vi "Chain2_bak.vi"(7 "Name (\"\" to Use UUID)":string="CSM-Module") -> ()   [LabVIEW 2017, in "CSM-Testcase.lvlib"]
doc: "Creates a template for a CSM module without a user interface.\n\n> [!NOTE] CSM Name Rules\n> - The CSM module name must be unique to avoid entering the \"Critical Error\" state.\n> - If the input is \"\", a UUID will be used as the module name. This module will operate in independent mode and will not be listed in the module list.\n> - If the input ends with '#', the module will run in work mode. Modules with the same name will share the same message queue. External messages will be handled by the idle module.\n\n> [!NOTE] CSM Initialization State\n> - The default value is \"Macro: Initialize\", consistent with the JKISM state machine.\n> - This state is typically not modified and is provided to facilitate external programmatic changes to the initialization state.\n\n\n-- <b>Controls</b> --\n- <b>Name (\"\" to Use UUID)</b>: CSM Module Name\n- <b>Init State(\"Macro: Initialize\")</b>: Initialization State, default is \"Macro: Initialize\""
uses:
  CSM-Testcase.lvlib
  250f9197-eaab-42aa-85f4-d19595f3ef40.vi
  b1f9a1d7-2f6f-40c5-bed8-42b286b8eb3f.vi
  e695532a-dccc-48b0-b567-f6fcd461bdfb.vi
  src/user.lib/_NEVSTOP/Communicable State Machine(CSM)/AdvanceAPI/CSM - Revert Arguments-Safe String.vi
  src/user.lib/_NEVSTOP/Communicable State Machine(CSM)/AdvanceAPI/CSM - Make String Arguments Safe.vi
  src/user.lib/_NEVSTOP/Communicable State Machine(CSM)/AdvanceAPI/CSM - Break Down Multiple States String.vi
  src/user.lib/_NEVSTOP/Communicable State Machine(CSM)/AdvanceAPI/CSM - Keywords.vi
  src/user.lib/_NEVSTOP/Communicable State Machine(CSM)/_Shared/Trim Single-line Text.vi
  Global-TestcaseCSM.vi
  src/user.lib/_NEVSTOP/Communicable State Machine(CSM)/_Polymophic/Build No-Reply Asynchronous Message with Arguments.vi
  src/user.lib/_NEVSTOP/Communicable State Machine(CSM)/_Polymophic/Build Asynchronous Message with Arguments.vi
  src/user.lib/_NEVSTOP/Communicable State Machine(CSM)/_Polymophic/Build Register Status Message.vi
  src/user.lib/_NEVSTOP/Communicable State Machine(CSM)/_Polymophic/Build Unregister Status Message.vi
  src/user.lib/_NEVSTOP/Communicable State Machine(CSM)/Communicable State Machine.lvlib
panel:
  out "Error Occurred":errorcluster
  out "State History":string
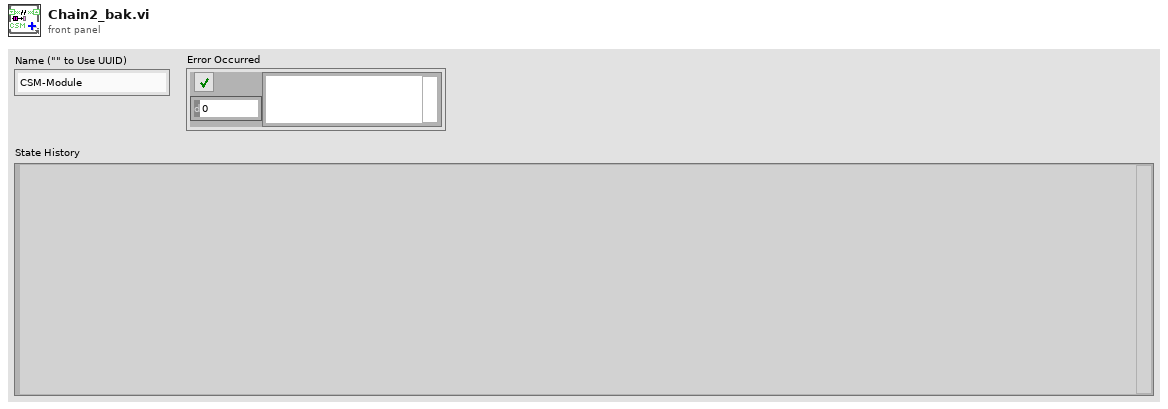
[diagram p1: front panel]
types:
  T1 = cluster{"Arguments":string, "Response":string, "error":errorcluster}
  T2 = enum32{"Invalid", "Standard", "Closed", "Hidden", "Minimized", "Maximized"}
  T3 = enum32{"invalid app kind", "Development System", "Run Time System", "Student Edition", "Embedded LabVIEW", "Evaluation", "Custom"}
  T4 = typedef "Communicable State Machine.lvlib/_CSM_Response Source Message.ctl" = cluster{"‘State":string, "’Arguments":string, "’Error":errorcluster}
  T5 = cluster{"Current VI Reference":refnum<vi>, "Close Panel on Exit?":bool}
  T6 = cluster{"Core":cluster{"Current VI Reference":refnum<vi>, "Close Panel on Exit?":bool}, "Your Boolean data":bool, "Your string data":string}
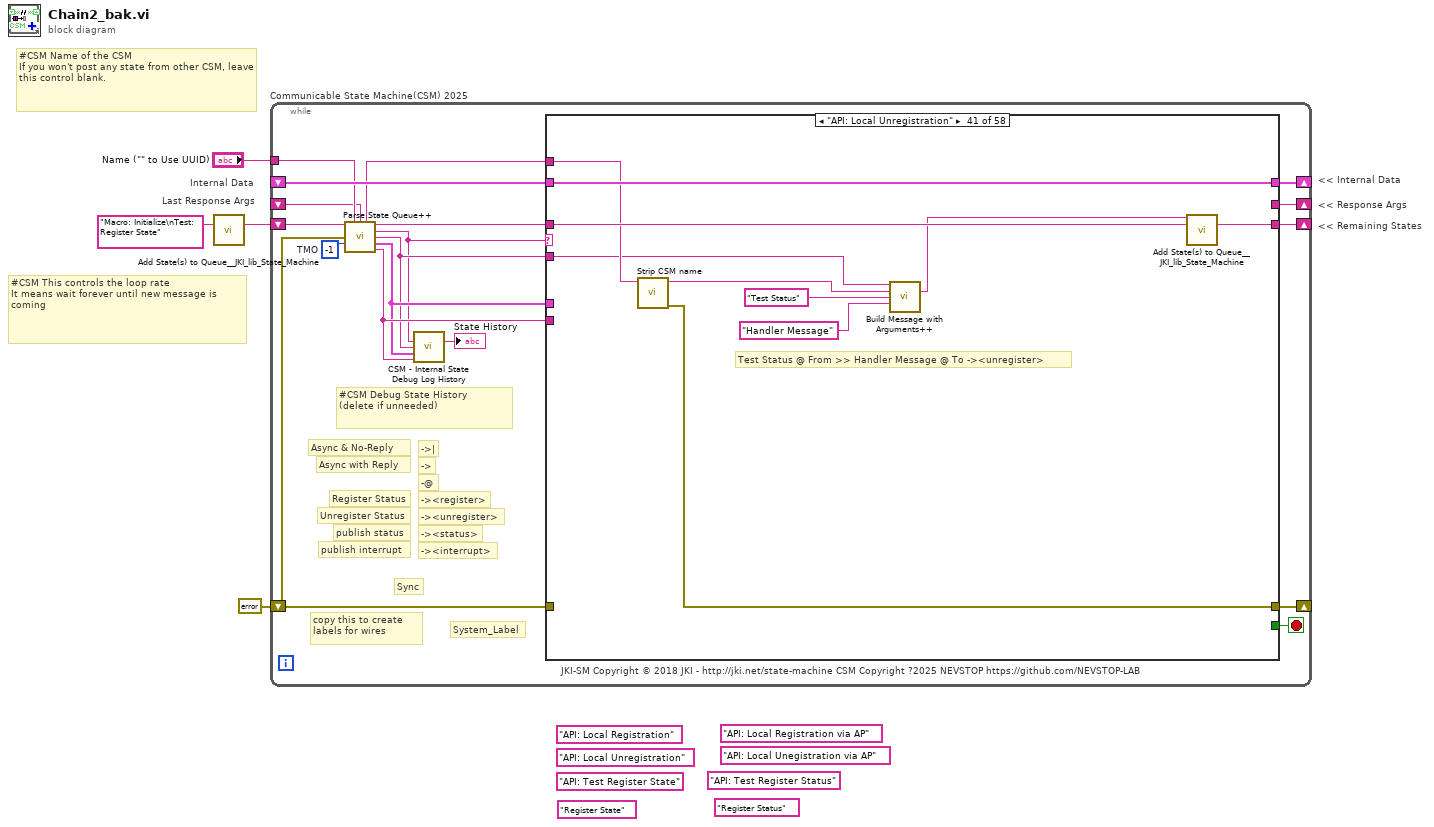
[diagram p0: block diagram]
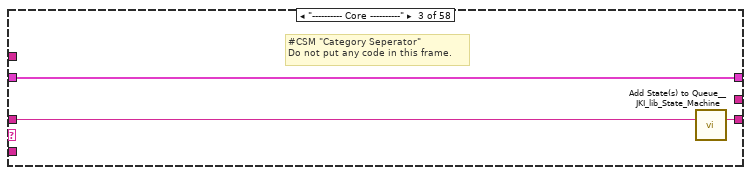
[diagram p4: hidden frame]
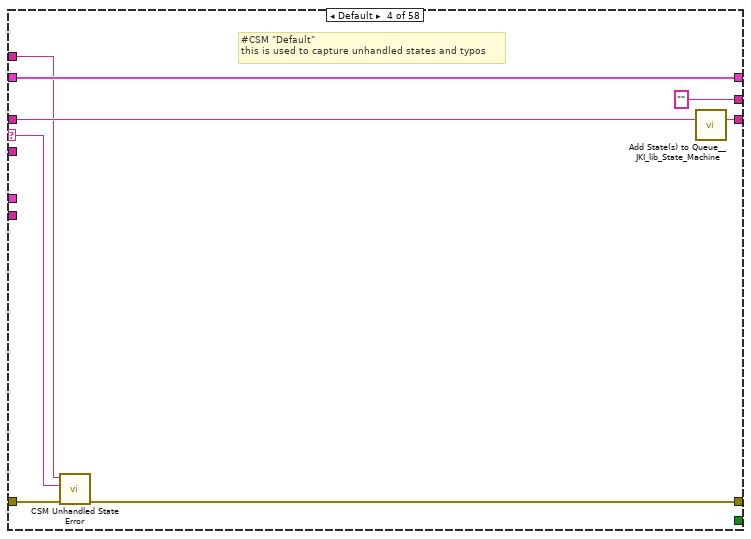
[diagram p5: hidden frame]
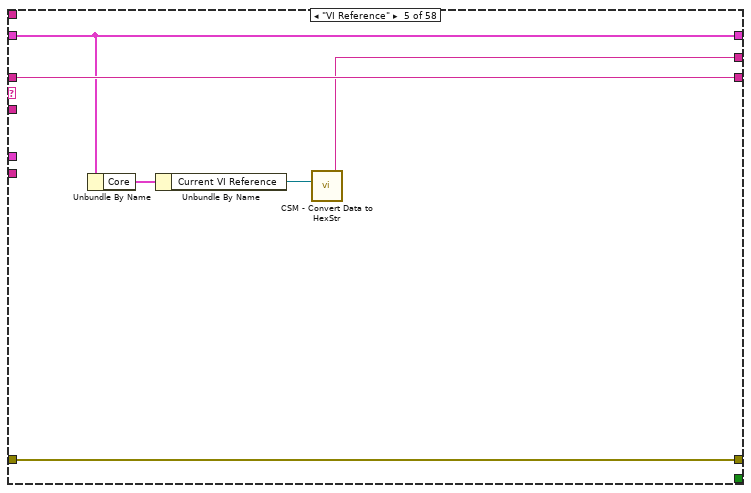
[diagram p6: hidden frame]
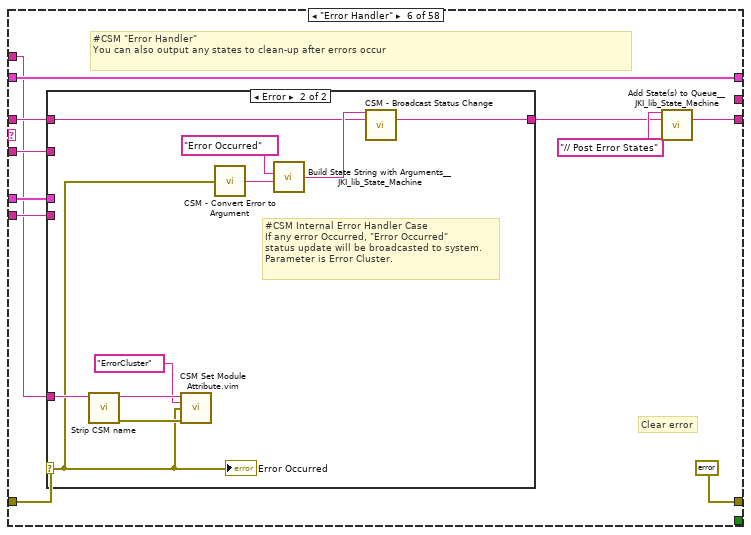
[diagram p7: hidden frame]
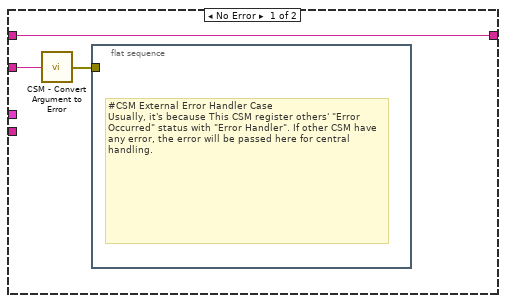
[diagram p8: hidden frame]
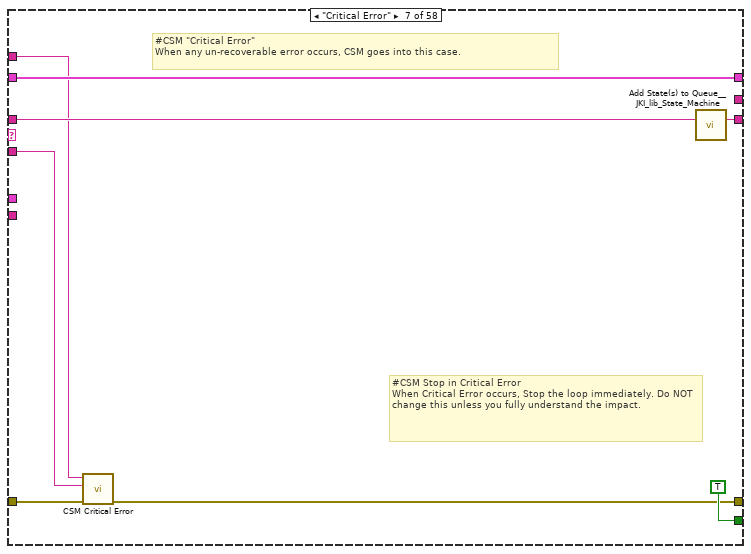
[diagram p9: hidden frame]
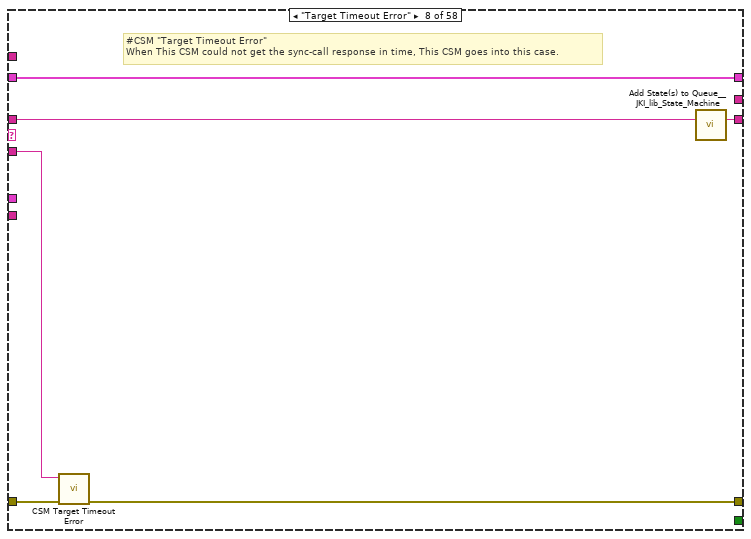
[diagram p10: hidden frame]
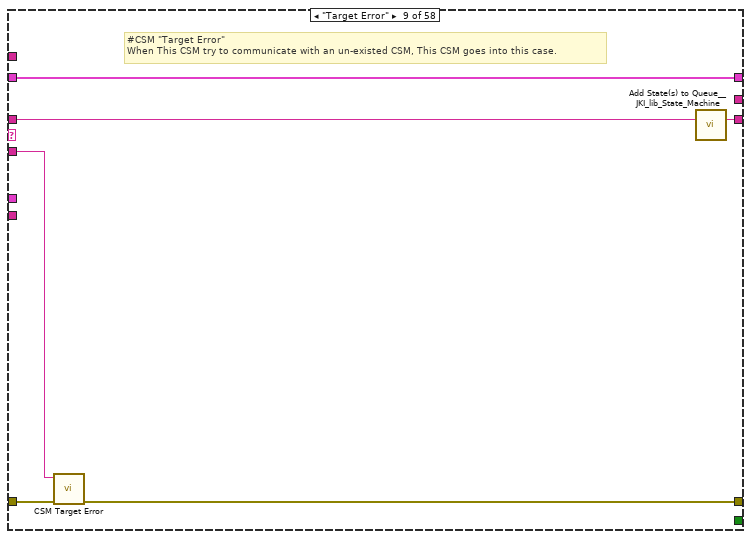
[diagram p11: hidden frame]
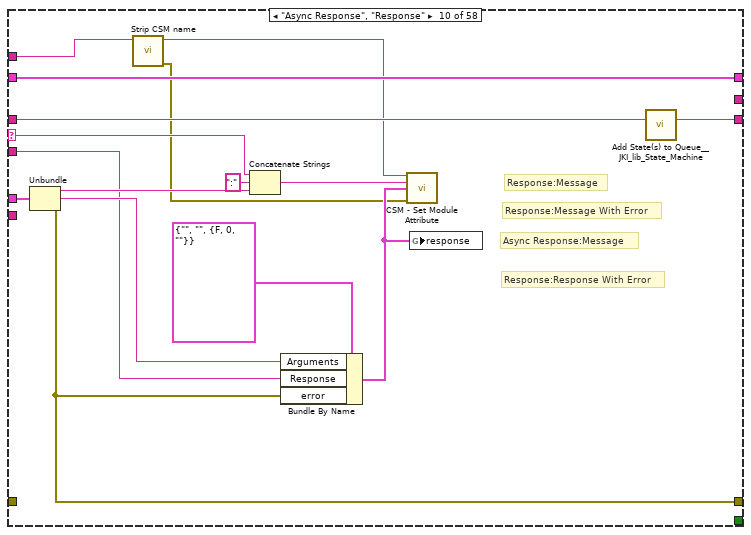
[diagram p12: hidden frame]
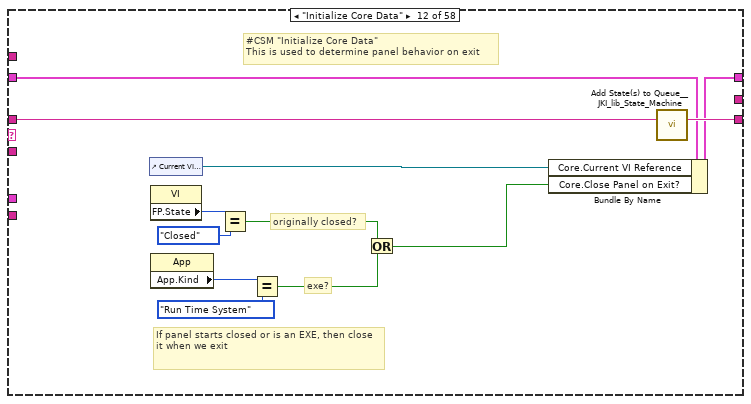
[diagram p14: hidden frame]
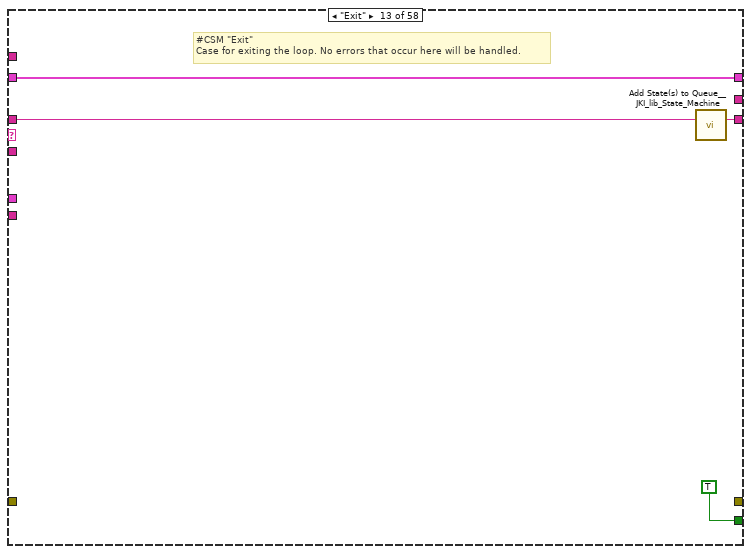
[diagram p15: hidden frame]
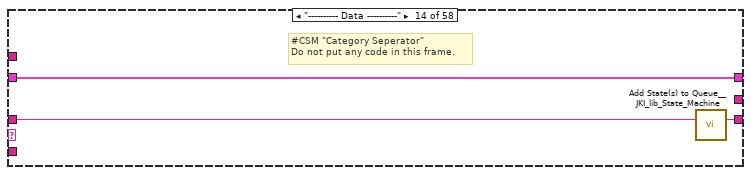
[diagram p16: hidden frame]
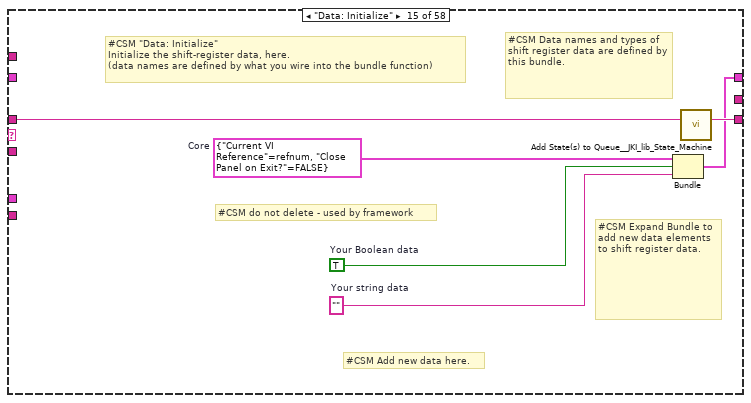
[diagram p17: hidden frame]
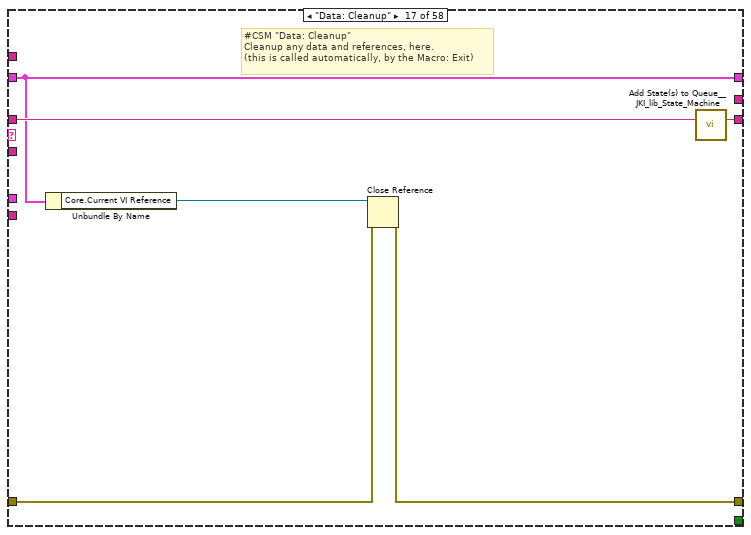
[diagram p19: hidden frame]
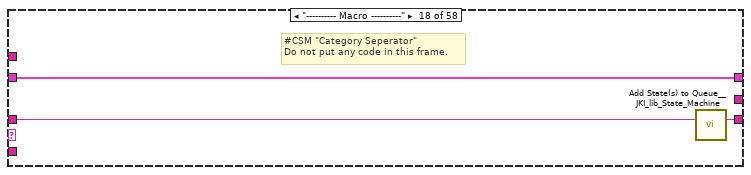
[diagram p20: hidden frame]
diagram:
  (unwired) "API: Local Unegistration via AP"
  (unwired) "API: Local Unregistration"
  (unwired) "API: Local Registration via AP"
  (unwired) "API: Local Registration"
  (unwired) "API: Test Register Status"
  (unwired) "API: Test Register State"
  (unwired) "Register State"
  (unwired) "Register Status"
  # "Last Response Args"
  # "Internal Data"
  # "#CSM Name of the CSM\nIf you won't post any state from other CSM, leave this control blank."
  # "#CSM This controls the loop rate\nIt means wait forever until new message is coming"
  # "<< Internal Data"
  # "<< Response Args"
  # "<< Remaining States"
  n1 = call <vilib>:"Add State(s) to Queue__JKI_lib_State_Machine.vi"("State(s) in (\"\")"="Macro: Initialize\nTest: Register State" ("Init State(\"Macro: Initialize\")")) -> ("States Out"=w4:string)  [unwired: 14 in]
  n2 = while "Communicable State Machine(CSM) 2025" {
    shift-right: [w17] -> _
    shift-left: _ -> [w16]
    shift-right: [w20] -> _
    shift-left: errorcluster {"status"=FALSE, "code"=0, "source"=""} ("error out") -> [w6]
    shift-right: [w19] -> _
    shift-left: w4 -> [w21]
    tunnel: "Name (\"\" to Use UUID)" -> [w13]
    shift-right: [w14] -> _
    shift-left: _ -> [w8]
    stop <- w18 stop-if-true
    w15 = -1  # TMO
    # "#CSM Debug State History\n(delete if unneeded)"
    # "-><interrupt>"
    # "-><status>"
    # "-><unregister>"
    # "-><register>"
    # "-@"
    # "->"
    # "->|"
    # "publish interrupt"
    # "publish status"
    # "Unregister Status"
    # "Register Status"
    # "Sync"
    # "Async with Reply"
    # "Async & No-Reply"
    # "JKI-SM Copyright © 2018 JKI - http://jki.net/state-machine CSM Copyright ?2025 NEVSTOP https://github.com/NEVSTOP-LAB"
    # "copy this to create labels for wires"
    # "System_Label"
    n3 = call "Parse State Queue++.vi"("State Queue"=w21, "Name (\"\" to Use UUID)"=w13, "Response Arguments"=w8, "Previous Error"=w6, "Dequeue (1 ms)"=w15) -> ("Name Used"=w7:string, "Remaining States"=w22:string, "Current State"=w9:string, "Arguments"=w10:string, ">> Response Source Message >>"=w11:T4, ">> Source CSM >>"=w12:string)  [unwired: 5 in]
    n4 = call "CSM - Internal State Debug Log History.vi"("State"=w9, "Arguments (\"\")"=w10, ">> Response Source Message >>"=w11, "Source (\"\")"=w12) -> ("Debug Log"=→"State History":string)  [unwired: 11 in]
    n5 = case shown="\"API: Local Unregistration\"" w9 {
      selector: w9 -> [_ _ _ w33 _ _ _ _ _ w99 _ _ _ _ _ _ _ _ _ _ _ _ _ _ _ _ _ _ _ _ _ _ _ _ _ _ _ _ _ _ _ _ _ _ _ _ _ _ _ _ _ w505 _ _ _ w530 w543 w549]
      tunnel: w22 -> [w23 w26 w29 w37 w42 w48 w75 w81 w87 w103 w105 w117 w121 w124 w130 w132 w138 w141 w145 w151 w165 w185 w214 w218 w222 w234 w262 w294 w310 w322 w334 w348 w371 w382 w395 w402 w409 w416 w423 w435 w445 w455 w465 w469 w474 w477 w483 w488 w491 w495 w499 w509 w513 w521 w527 w535 w545 w555]
      tunnel: w10 -> [_ _ _ _ _ w47 w71 w78 w84 w93 _ _ _ _ _ _ _ _ _ _ w152 w172 w197 _ w225 w237 w265 w297 w313 w325 w337 w351 w367 w385 w392 w399 w406 w413 w420 w427 w437 w446 w456 w467 _ _ w479 w484 w490 w494 w498 w504 w512 w519 w525 w532 w544 w548]
      tunnel: w16 -> [w24 w25 w27 w35 w41 w53 w73 w79 w85 w101 w104 w111 w119 w122 _ w131 w133 w139 w143 w149 w167 w187 w216 w217 w226 w238 w266 w298 w314 w326 w338 w352 w374 w386 w397 w404 w411 w418 w425 w433 w443 w453 w463 w468 w472 w475 w481 w489 w492 w496 w500 w510 w514 w520 w526 w536 w546 w556]
      tunnel: [_ _ _ w30 w43 errorcluster {"status"=FALSE, "code"=0, "source"=""} ("error out") w68 w76 w82 w92 _ _ _ _ _ _ w134 _ _ _ _ _ _ _ w219 w231 w259 w291 w307 w319 w331 w344 w368 w379 w396 w403 w410 w417 w424 w429 w439 w450 w460 _ _ _ _ _ w493 w497 w501 w503 w515 w516 w522 w529 w539 w551] -> w20
      tunnel: w6 -> [_ _ _ w31 w43 w51 w69 w77 w83 _ _ _ _ _ _ _ w135 _ _ _ _ _ _ _ _ _ _ _ _ _ _ _ _ _ w396 w403 w410 w417 w424 _ _ _ _ _ _ _ _ _ w493 w497 w501 w511 w515 w517 w523 w537 w547 w557]
      tunnel: [w23 w26 w28 w36 w42 w49 w74 w80 w86 w102 w105 w116 w120 w123 w129 w132 w137 w140 w144 w150 w166 w186 w215 w218 w223 w235 w263 w295 w311 w323 w335 w349 w372 w383 w394 w401 w408 w415 w422 w434 w444 w454 w464 w469 w473 w476 w482 w485 w491 w495 w499 w509 w513 w521 w527 w535 w545 w555] -> w19
      tunnel: [_ _ _ _ _ _ TRUE _ _ _ _ _ TRUE _ _ _ _ _ _ _ _ _ _ _ _ _ _ _ _ _ _ _ _ _ _ _ _ _ _ _ _ _ _ _ _ _ _ _ _ _ _ _ _ _ _ _ _ _] -> w18
      tunnel: [w24 w25 w27 w35 w41 w53 w73 w79 w85 w101 w104 w115 w119 w122 w128 w131 w133 w139 w143 w149 w167 w187 w216 w217 w226 w238 w266 w298 w314 w326 w338 w352 w374 w386 w397 w404 w411 w418 w425 w433 w443 w453 w463 w468 w472 w475 w481 w489 w492 w496 w500 w510 w514 w520 w526 w536 w546 w556] -> w17
      tunnel: w12 -> [_ _ _ _ _ w46 _ _ _ _ _ _ _ _ _ _ _ _ _ _ _ _ _ _ _ _ _ _ _ _ _ _ _ _ _ _ _ _ _ _ _ _ _ _ _ _ _ _ _ _ _ _ _ _ _ _ _ _]
      tunnel: w11 -> [_ _ _ _ _ w45 _ _ _ w100 _ _ _ _ _ _ _ _ _ _ _ _ _ _ _ _ _ _ _ _ _ _ _ _ _ _ _ _ _ _ _ _ _ _ _ _ _ _ _ _ _ _ _ _ _ _ _ _]
      tunnel: [_ _ _ "" w38 _ _ _ _ _ _ _ _ _ _ _ _ _ _ _ _ _ _ _ _ _ _ _ _ _ _ _ _ _ _ _ _ _ _ _ _ _ _ w466 _ _ _ _ w490 w494 w498 w504 w512 w519 w525 _ w544 w548] -> w14
      tunnel: w7 -> [_ _ _ w32 _ w44 w70 _ _ w90 _ _ _ _ _ _ _ _ _ _ _ _ _ _ _ _ w250 w282 _ _ _ w345 _ _ _ _ _ _ _ w431 w441 w452 w462 _ _ _ _ _ _ _ _ w508 _ _ _ w534 w542 w554]
      frame "", "Idle" {
        # "#CSM \"Idle/Event Handler\"\nexecutes when the state queue is empty"
      }
      frame "CSM Documentation" {
        # "#CSM State Syntax\n\n// Comment line, all text to the right of “//” will be ignored\n// Local Message Example\nDoSth: DoA >> Arguments\n\n// Sync Call Example\nAPI: xxxx >> Arguments -@ TargetModule\n\n// Async Call Example\nAPI: xxxx >> Arguments -> TargetModule\n\n// Async Call without Reply Example\nAPI: xxxx >> Arguments ->| TargetModule\n\n// Broadcast normal status:\nStatus >> StatusArguments  -><status>\n\n// Broadcast Interrupt status:\nInterrupt >> StatusArguments  -><interrupt>\n\n// Register Source Module's status to Handler Module\nStatus@Source Module >> Handler Module@Handler Module -><register>\n\n// Unegister Source Module's status\nStatus@Source Module >> Handler Module -><unregister>"
        # "#CSM README FIRST\n\nCommunicable State Machine(CSM) is a LabVIEW application framework that builds upon JKI State Machine(JKISM). It follows the pattern of JKISM and extends the keywords to describe message communication between modules, including concepts such as Sync-Message, Async-Message, Subscription/Unsubscription of status - essential elements for creating reusable code modules. For more information, please visit the CSM wiki: https://nevstop-lab.github.io/CSM-Wiki/\n\nFor instructions on JKI State Machine, visit: \n    http://jki.net/state-machine/\nFor information about CSM, visit: \n    https://github.com/NEVSTOP-LAB"
        # "#CSM \"Documentation\"\nCase for holding CSM Documenation"
      }
      frame "---------- Core ----------" {
        # "#CSM \"Category Seperator\"\nDo not put any code in this frame."
        n6 = call <vilib>:"Add State(s) to Queue__JKI_lib_State_Machine.vi"("State(s) in (\"\")"=w29) -> ("States Out"=w28:string)  [unwired: 14 in]
      }
      frame Default {
        # "#CSM \"Default\"\nthis is used to capture unhandled states and typos"
        n7 = call "CSM Unhandled State Error.vi"("error in (no error)"=w31, "Current State"=w33, "CSM Name"=w32) -> ("error out"=w30:errorcluster)  [unwired: 8 in]
        n8 = call <vilib>:"Add State(s) to Queue__JKI_lib_State_Machine.vi"("State(s) in (\"\")"=w37) -> ("States Out"=w36:string)  [unwired: 14 in]
      }
      frame "VI Reference" {
        n9 = Unbundle By Name(w41) -> ("Core"=w40:T5)
        n10 = Unbundle By Name(w40) -> ("Current VI Reference"=w39:refnum<vi>)
        n11 = call "CSM - Convert Data to HexStr.vi"("Variant"=w39) -> ("HEX String (0-9,A-F)"=w38:string)  [unwired: 8 in]
      }
      frame "Error Handler" {
        # "#CSM \"Error Handler\"\nYou can also output any states to clean-up after errors occur"
        # "Clear error"
        n12 = case shown="Error" w51 {
          selector: w51 -> [_ w59]
          tunnel: [w57 w64] -> w50
          tunnel: w48 -> [w57 w63]
          tunnel: w47 -> [w56 _]
          tunnel: w46 -> [_ _]
          tunnel: w45 -> [_ _]
          tunnel: w44 -> [_ w62]
          frame No Error {
            n13 = call "CSM - Convert Argument to Error.vi"("Argument"=w56) -> ("Error"=w55:errorcluster)  [unwired: 4 in]
            n14 = flat-sequence {
              tunnel: w55 -> [_]
              frame #0 {
                # "#CSM External Error Handler Case\nUsually, it's because This CSM register others' \"Error Occurred\" status with \"Error Handler\". If other CSM have any error, the error will be passed here for central handling."
              }
            }
          }
          frame Error {
            # "#CSM Internal Error Handler Case \nIf any error Occurred, \"Error Occurred\" \nstatus update will be broadcasted to system.\nParameter is Error Cluster."
            n15 = call "Strip CSM name.vi"("CSM name"=w62) -> ("error out"=w61:errorcluster, "CSM name core"=w60:string)  [unwired: 7 in, 2 out]
            n16 = call "CSM Set Module Attribute.vim"("CSM Name"=w60, "Attribute"="ErrorCluster", "Value"=w59, "Error In"=w61) -> ()  [unwired: 8 in, 4 out]
            n17 = call "CSM - Convert Error to Argument.vi"("Error"=w59) -> ("Argument"=w66:string)  [unwired: 4 in]
            n18 = call <vilib>:"Build State String with Arguments__JKI_lib_State_Machine.vi"("Arguments (\"\")"=w66, "State"="Error Occurred" ("Status with Arguments")) -> ("State with Arguments"=w65:string)  [unwired: 4 in]
            n19 = call "CSM - Broadcast Status Change.vi"("Status With Arguments"=w65, "State Queue"=w63) -> ("Remaining States"=w64:string)  [unwired: 13 in]
            "Error Occurred" <- w59
          }
        }
        n20 = call <vilib>:"Add State(s) to Queue__JKI_lib_State_Machine.vi"("State(s) in Front (\"\")"="// Post Error States", "State(s) in (\"\")"=w50) -> ("States Out"=w49:string)  [unwired: 13 in]
      }
      frame "Critical Error" {
        # "#CSM \"Critical Error\"\nWhen any un-recoverable error occurs, CSM goes into this case."
        # "#CSM Stop in Critical Error\nWhen Critical Error occurs, Stop the loop immediately. Do NOT change this unless you fully understand the impact."
        n21 = call "CSM Critical Error.vi"("error in (no error)"=w69, "Arugments (As Reason)"=w71, "CSM Name"=w70) -> ("error out"=w68:errorcluster)  [unwired: 8 in]
        n22 = call <vilib>:"Add State(s) to Queue__JKI_lib_State_Machine.vi"("State(s) in (\"\")"=w75) -> ("States Out"=w74:string)  [unwired: 14 in]
      }
      frame "Target Timeout Error" {
        # "#CSM \"Target Timeout Error\"\nWhen This CSM could not get the sync-call response in time, This CSM goes into this case."
        n23 = call "CSM Target Timeout Error.vi"("error in (no error)"=w77, "Arguments (As CSM Name)"=w78) -> ("error out"=w76:errorcluster)  [unwired: 9 in]
        n24 = call <vilib>:"Add State(s) to Queue__JKI_lib_State_Machine.vi"("State(s) in (\"\")"=w81) -> ("States Out"=w80:string)  [unwired: 14 in]
      }
      frame "Target Error" {
        # "#CSM \"Target Error\"\nWhen This CSM try to communicate with an un-existed CSM, This CSM goes into this case."
        n25 = call "CSM Target Error.vi"("error in (no error)"=w83, "Arguments (As CSM Name)"=w84) -> ("error out"=w82:errorcluster)  [unwired: 9 in]
        n26 = call <vilib>:"Add State(s) to Queue__JKI_lib_State_Machine.vi"("State(s) in (\"\")"=w87) -> ("States Out"=w86:string)  [unwired: 14 in]
      }
      frame "Async Response", "Response" {
        # "Response:Response With Error"
        # "Response:Message With Error"
        # "Async Response:Message"
        # "Response:Message"
        n27 = Unbundle(w100) -> ("‘State"=w98:string, "’Arguments"=w94:string, "’Error"=w92:errorcluster)
        n28 = call "Strip CSM name.vi"("CSM name"=w90) -> ("error out"=w88:errorcluster, "CSM name core"=w89:string)  [unwired: 7 in, 2 out]
        n29 = Concatenate Strings(w99, ":" ("string"), w98) -> (w96:string)
        n30 = Bundle By Name(cluster=T1 {"Arguments"="", "Response"="", "error"={"status"=FALSE, "code"=0, "source"=""}}, "Arguments"=w94, "Response"=w93, "error"=w92) -> (w91:T1)
        n31 = call "CSM - Set Module Attribute.vi"("CSM Name"=w89, "Attribute"=w96, "Value"=w91, "Error In"=w88) -> ()  [unwired: 8 in, 4 out]
        n32 = global write "Global-TestcaseCSM.vi" "response"(w91) -> ()
        n33 = call <vilib>:"Add State(s) to Queue__JKI_lib_State_Machine.vi"("State(s) in (\"\")"=w103) -> ("States Out"=w102:string)  [unwired: 14 in]
      }
      frame "Async Message Posted" {
        # "#CSM \"Async Message Posted\"\nAfter Async Message is posted (-> or ->| ), CSM goes to this state for post-action.\nYou can use Argument - State to tell which Async Message is called."
      }
      frame "Initialize Core Data" {
        # "#CSM \"Initialize Core Data\"\nThis is used to determine panel behavior on exit"
        # "originally closed?"
        # "exe?"
        # "If panel starts closed or is an EXE, then close it when we exit"
        n34 = control-ref of="Current VI Reference"() -> (w109:refnum<vi>)
        n35 = property class="VI"() -> ("FP.State"=w108:T2)  [unwired: 2 in, 2 out]
        n36 = property class="App"() -> ("App.Kind"=w114:T3)  [unwired: 2 in, 2 out]
        n37 = Equal?(x=w108, y=T2."Closed" ("Front Panel Window:State")) -> (x = y?=w106:bool)
        n38 = Equal?(x=w114, y=T3."Run Time System" ("Application:Kind")) -> (x = y?=w112:bool)
        n39 = Or(x=w106, y=w112) -> (x .or. y?=w110:bool)
        n40 = Bundle By Name(cluster=w111, "Core.Current VI Reference"=w109, "Core.Close Panel on Exit?"=w110) -> (w115:T6)
        n41 = call <vilib>:"Add State(s) to Queue__JKI_lib_State_Machine.vi"("State(s) in (\"\")"=w117) -> ("States Out"=w116:string)  [unwired: 14 in]
      }
      frame "Exit" {
        # "#CSM \"Exit\"\nCase for exiting the loop. No errors that occur here will be handled."
        n42 = call <vilib>:"Add State(s) to Queue__JKI_lib_State_Machine.vi"("State(s) in (\"\")"=w121) -> ("States Out"=w120:string)  [unwired: 14 in]
      }
      frame "---------- Data ----------" {
        # "#CSM \"Category Seperator\"\nDo not put any code in this frame."
        n43 = call <vilib>:"Add State(s) to Queue__JKI_lib_State_Machine.vi"("State(s) in (\"\")"=w124) -> ("States Out"=w123:string)  [unwired: 14 in]
      }
      frame "Data: Initialize" {
        w125 = T5 {"Current VI Reference"=refnum, "Close Panel on Exit?"=FALSE}  # Core
        w127 = TRUE  # Your Boolean data
        w126 = ""  # Your string data
        # "#CSM \"Data: Initialize\"\nInitialize the shift-register data, here.\n(data names are defined by what you wire into the bundle function)"
        # "#CSM do not delete - used by framework"
        # "#CSM Expand Bundle to add new data elements to shift register data."
        # "#CSM Add new data here."
        # "#CSM Data names and types of shift register data are defined by this bundle."
        n44 = Bundle("Core"=w125, "Your Boolean data"=w127, "Your string data"=w126) -> (w128:T6)  [unwired: 1 in]
        n45 = call <vilib>:"Add State(s) to Queue__JKI_lib_State_Machine.vi"("State(s) in (\"\")"=w130) -> ("States Out"=w129:string)  [unwired: 14 in]
      }
      frame "Data: Update Indicators" {
      }
      frame "Data: Cleanup" {
        # "#CSM \"Data: Cleanup\"\nCleanup any data and references, here.\n(this is called automatically, by the Macro: Exit)"
        n46 = Unbundle By Name(w133) -> ("Core.Current VI Reference"=w136:refnum<vi>)
        n47 = Close Reference(reference=w136, error in (no error)=w135) -> (error out=w134:errorcluster)
        n48 = call <vilib>:"Add State(s) to Queue__JKI_lib_State_Machine.vi"("State(s) in (\"\")"=w138) -> ("States Out"=w137:string)  [unwired: 14 in]
      }
      frame "---------- Macro ----------" {
        # "#CSM \"Category Seperator\"\nDo not put any code in this frame."
        n49 = call <vilib>:"Add State(s) to Queue__JKI_lib_State_Machine.vi"("State(s) in (\"\")"=w141) -> ("States Out"=w140:string)  [unwired: 14 in]
      }
      frame "Macro: Initialize" {
        # "#CSM \"Macro: Initialize\"\nInitialization Macro (This is called once, when the VI starts)"
        n50 = call <vilib>:"Add State(s) to Queue__JKI_lib_State_Machine.vi"("State(s) in Front (\"\")"="Data: Initialize\nInitialize Core Data\nData: Update Indicators", "State(s) in (\"\")"=w145) -> ("States Out"=w144:string)  [unwired: 13 in]
      }
      frame "Macro: Exit" {
        # "#CSM \"Macro: Exit\"\nExit Macro (This is called once, when the VI exits)"
        n51 = call <vilib>:"Add State(s) to Queue__JKI_lib_State_Machine.vi"("State(s) in Front (\"\")"="//Exit Sub-Modules ", "State(s) at Back (\"\")"="Data: Cleanup\nExit") -> ("States Out"=w147:string)  [unwired: 13 in]
        n52 = call <vilib>:"Add State(s) to Queue__JKI_lib_State_Machine.vi"("State(s) in Front (\"\")"=w147, "State(s) in (\"\")"=w151) -> ("States Out"=w150:string)  [unwired: 13 in]
      }
      frame "Macro: Test MacroWithSubMessages" {
        w153 = "SubMessage2" ("State With Arguments")
        w155 = "SubMessage1" ("State With Arguments")
        n53 = call "uuid.vi"() -> ("UUID"=w154:string)  [unwired: 11 in]
        n54 = call "uuid.vi"() -> ("UUID"=w156:string)  [unwired: 11 in]
        n55 = Concatenate Strings(w155, w156) -> (w157:string)
        n56 = Concatenate Strings(w153, w154) -> (w158:string)
        n57 = call <vilib>:"Build State String with Arguments__JKI_lib_State_Machine.vi"("Arguments (\"\")"=w152, "State"="SubMessage3" ("State With Arguments")) -> ("State with Arguments"=w160:string)  [unwired: 4 in]
        n58 = call <vilib>:"Build State String with Arguments__JKI_lib_State_Machine.vi"("Arguments (\"\")"=w157, "State"=w155) -> ("State with Arguments"=w162:string)  [unwired: 4 in]
        n59 = call <vilib>:"Build State String with Arguments__JKI_lib_State_Machine.vi"("Arguments (\"\")"=w158, "State"=w153) -> ("State with Arguments"=w161:string)  [unwired: 4 in]
        n60 = Build Array(w162, w161, w160) -> (w159:string[])
        n61 = call "CSM - Compact Multiple States.vi"("Multiple States"=w159) -> ("States"=w164:string)  [unwired: 9 in]
        n62 = call <vilib>:"Add State(s) to Queue__JKI_lib_State_Machine.vi"("State(s) in Front (\"\")"=w164, "State(s) in (\"\")"=w165) -> ("States Out"=w166:string)  [unwired: 13 in]
      }
      frame "Macro: Test MacroWithSubAndPostMessages" {
        w171 = "PostMessage1" ("State With Arguments")
        w173 = "SubMessage2" ("State With Arguments")
        w175 = "SubMessage1" ("State With Arguments")
        n63 = call "uuid.vi"() -> ("UUID"=w174:string)  [unwired: 11 in]
        n64 = call "uuid.vi"() -> ("UUID"=w170:string)  [unwired: 11 in]
        n65 = call "uuid.vi"() -> ("UUID"=w176:string)  [unwired: 11 in]
        n66 = Concatenate Strings(w171, w170) -> (w169:string)
        n67 = Concatenate Strings(w175, w176) -> (w177:string)
        n68 = Concatenate Strings(w173, w174) -> (w178:string)
        n69 = call <vilib>:"Build State String with Arguments__JKI_lib_State_Machine.vi"("Arguments (\"\")"=w172, "State"="SubMessage3" ("State With Arguments")) -> ("State with Arguments"=w180:string)  [unwired: 4 in]
        n70 = call <vilib>:"Build State String with Arguments__JKI_lib_State_Machine.vi"("Arguments (\"\")"=w169, "State"=w171) -> ("State with Arguments"=w168:string)  [unwired: 4 in]
        n71 = call <vilib>:"Build State String with Arguments__JKI_lib_State_Machine.vi"("Arguments (\"\")"=w177, "State"=w175) -> ("State with Arguments"=w182:string)  [unwired: 4 in]
        n72 = call <vilib>:"Build State String with Arguments__JKI_lib_State_Machine.vi"("Arguments (\"\")"=w178, "State"=w173) -> ("State with Arguments"=w181:string)  [unwired: 4 in]
        n73 = Build Array(w182, w181, w180) -> (w179:string[])
        n74 = call "CSM - Compact Multiple States.vi"("Multiple States"=w179) -> ("States"=w184:string)  [unwired: 9 in]
        n75 = call <vilib>:"Add State(s) to Queue__JKI_lib_State_Machine.vi"("State(s) in Front (\"\")"=w184, "State(s) in (\"\")"=w185, "State(s) at Back (\"\")"=w168) -> ("States Out"=w186:string)  [unwired: 12 in]
      }
      frame "Macro: TestMacroWithNonLocalSubMessages" {
        w201 = "PostMessage1" ("State With Arguments")
        w202 = "SubMessage2" ("State With Arguments")
        w204 = "SubMessage1" ("State With Arguments")
        n76 = Match Pattern(string=w197, regular expression="+") -> (before substring=w189:string, after substring=w188:string)  [unwired: 1 in, 2 out]
        n77 = call "uuid.vi"() -> ("UUID"=w200:string)  [unwired: 11 in]
        n78 = call "uuid.vi"() -> ("UUID"=w203:string)  [unwired: 11 in]
        n79 = call "uuid.vi"() -> ("UUID"=w205:string)  [unwired: 11 in]
        n80 = Concatenate Strings(w201, w200) -> (w199:string)
        n81 = Concatenate Strings(w204, w205) -> (w206:string)
        n82 = Concatenate Strings(w202, w203) -> (w207:string)
        n83 = call <vilib>:"Build State String with Arguments__JKI_lib_State_Machine.vi"("Arguments (\"\")"=w199, "State"=w201) -> ("State with Arguments"=w198:string)  [unwired: 4 in]
        n84 = call-poly "Build Message with Arguments++.vi"("State With Arguments"="SubMessage1", "Target Module (\"\")"=w188) -> ("CSM Message String"=w193:string)  [unwired: 13 in]
        n85 = call-poly "Build Message with Arguments++.vi"("State With Arguments"="SubMessage2", "Target Module (\"\")"=w188) -> ("CSM Message String"=w192:string)  [unwired: 13 in]
        n86 = call <vilib>:"Build State String with Arguments__JKI_lib_State_Machine.vi"("Arguments (\"\")"=w189, "State"="SubMessage3" ("State With Arguments")) -> ("State with Arguments"=w209:string)  [unwired: 4 in]
        n87 = call-poly "Build Message with Arguments++.vi"("State With Arguments"="Message", "Target Module (\"\")"=w188) -> ("CSM Message String"=w194:string)  [unwired: 13 in]
        n88 = call <vilib>:"Build State String with Arguments__JKI_lib_State_Machine.vi"("Arguments (\"\")"=w206, "State"=w204) -> ("State with Arguments"=w211:string)  [unwired: 4 in]
        n89 = call <vilib>:"Build State String with Arguments__JKI_lib_State_Machine.vi"("Arguments (\"\")"=w207, "State"=w202) -> ("State with Arguments"=w210:string)  [unwired: 4 in]
        n90 = Build Array(w211, w210, w209, w194, w193, w192) -> (w208:string[])
        n91 = call "CSM - Compact Multiple States.vi"("Multiple States"=w208) -> ("States"=w213:string)  [unwired: 9 in]
        n92 = call <vilib>:"Add State(s) to Queue__JKI_lib_State_Machine.vi"("State(s) in Front (\"\")"=w213, "State(s) in (\"\")"=w214, "State(s) at Back (\"\")"=w198) -> ("States Out"=w215:string)  [unwired: 12 in]
      }
      frame "---------- API ----------" {
        # "#CSM \"Category Seperator\"\nDo not put any code in this frame."
      }
      frame "API: Test SyncMessage" {
        n93 = call "CSM - Check If Module Exists.vi"("CSM Name"=w225) -> ("error out"=w219:errorcluster, "Exist?"=w220:bool, "CSM Name (Dup)"=w224:string)  [unwired: 8 in]
        n94 = case shown="True" w220 {
          tunnel: w224 -> [_ w228]
          tunnel: [_ w227] -> w221
          frame False {
          }
          frame True {
            n95 = call "uuid.vi"() -> ("UUID"=w229:string)  [unwired: 11 in]
            n96 = call "Build Synchronous Message with Arguments.vi"("State With Arguments"="Message", "Arguments (\"\")"=w229, "Target Module (\"\")"=w228) -> ("CSM Message String"=w227:string)  [unwired: 12 in]
          }
        }
        n97 = call <vilib>:"Add State(s) to Queue__JKI_lib_State_Machine.vi"("State(s) in Front (\"\")"=w221, "State(s) in (\"\")"=w222) -> ("States Out"=w223:string)  [unwired: 13 in]
      }
      frame "API: Test SyncMessage With Error" {
        n98 = call "CSM - Check If Module Exists.vi"("CSM Name"=w237) -> ("error out"=w231:errorcluster, "Exist?"=w232:bool, "CSM Name (Dup)"=w236:string)  [unwired: 8 in]
        n99 = case shown="True" w232 {
          tunnel: w236 -> [_ w240]
          tunnel: [_ w239] -> w233
          frame False {
          }
          frame True {
            n100 = call "uuid.vi"() -> ("UUID"=w241:string)  [unwired: 11 in]
            n101 = call "Build Synchronous Message with Arguments.vi"("State With Arguments"="Message With Error", "Arguments (\"\")"=w241, "Target Module (\"\")"=w240) -> ("CSM Message String"=w239:string)  [unwired: 12 in]
          }
        }
        n102 = call <vilib>:"Add State(s) to Queue__JKI_lib_State_Machine.vi"("State(s) in Front (\"\")"=w233, "State(s) in (\"\")"=w234) -> ("States Out"=w235:string)  [unwired: 13 in]
      }
      frame "API: Test SyncMessage via API" {
        n103 = call "CSM - Check If Module Exists.vi"("CSM Name"=w265) -> ("error out"=w260:errorcluster, "Exist?"=w261:bool, "CSM Name (Dup)"=w264:string)  [unwired: 8 in]
        n104 = case shown="True" w261 {
          tunnel: w264 -> [_ w274]
          tunnel: [_ w273] -> w248
          tunnel: w250 -> [_ w272]
          tunnel: [_ w271] -> w257
          tunnel: [_ w270] -> w246
          tunnel: [_ w269] -> w253
          tunnel: [_ w268] -> w256
          frame False {
          }
          frame True {
            w271 = "Message" ("State With Arguments")
            n105 = call "uuid.vi"() -> ("UUID"=w269:string)  [unwired: 11 in]
            n106 = call "CSM - Wait and Send Message for Reply.vi"("State"=w271, "Current Module (\"\" to Generate an ID)"=w272, "Arguments (\"\")"=w269, "Target Module"=w274) -> ("Response"=w268:string, ">> Source CSM >>"=w270:string, "error out"=w273:errorcluster)  [unwired: 9 in]
          }
        }
        n107 = call "Strip CSM name.vi"("CSM name"=w250) -> ("error out"=w247:errorcluster, "CSM name core"=w249:string)  [unwired: 7 in, 2 out]
        n108 = call "Strip CSM name.vi"("CSM name"=w246) -> ("error out"=w243:errorcluster, "CSM name core"=w245:string)  [unwired: 7 in, 2 out]
        n109 = Bundle By Name(cluster=T1 {"Arguments"="", "Response"="", "error"={"status"=FALSE, "code"=0, "source"=""}}, "Arguments"=w253, "Response"=w256, "error"=w248) -> (w251:T1)
        n110 = Concatenate Strings(w245, ":" ("string"), w257) -> (w255:string)
        n111 = Merge Errors(w247, w243) -> (w244:errorcluster)
        n112 = call "CSM - Set Module Attribute.vi"("CSM Name"=w249, "Attribute"=w255, "Value"=w251, "Error In"=w244) -> ("error out"=w254:errorcluster)  [unwired: 8 in, 3 out]
        n113 = disable-structure shown="Enabled" {
          disable-tunnel: w251 -> [w267 _]
          frame Enabled {
            n114 = global write "Global-TestcaseCSM.vi" "response"(w267) -> ()
          }
          frame Disabled {
          }
        }
        n115 = call <vilib>:"Add State(s) to Queue__JKI_lib_State_Machine.vi"("State(s) in (\"\")"=w262) -> ("States Out"=w263:string)  [unwired: 14 in]
        n116 = Merge Errors(w254, w248, w260) -> (w259:errorcluster)
      }
      frame "API: Test SyncMessage With Error via API" {
        n117 = call "CSM - Check If Module Exists.vi"("CSM Name"=w297) -> ("error out"=w292:errorcluster, "Exist?"=w293:bool, "CSM Name (Dup)"=w296:string)  [unwired: 8 in]
        n118 = case shown="True" w293 {
          tunnel: w296 -> [_ w306]
          tunnel: [_ w305] -> w279
          tunnel: w282 -> [_ w304]
          tunnel: [_ w303] -> w289
          tunnel: [_ w302] -> w278
          tunnel: [_ w301] -> w285
          tunnel: [_ w300] -> w288
          frame False {
          }
          frame True {
            w303 = "Message With Error" ("State With Arguments")
            n119 = call "uuid.vi"() -> ("UUID"=w301:string)  [unwired: 11 in]
            n120 = call "CSM - Wait and Send Message for Reply.vi"("State"=w303, "Current Module (\"\" to Generate an ID)"=w304, "Arguments (\"\")"=w301, "Target Module"=w306) -> ("Response"=w300:string, ">> Source CSM >>"=w302:string, "error out"=w305:errorcluster)  [unwired: 9 in]
          }
        }
        n121 = call "Strip CSM name.vi"("CSM name"=w278) -> ("error out"=w275:errorcluster, "CSM name core"=w277:string)  [unwired: 7 in, 2 out]
        n122 = Bundle By Name(cluster=T1 {"Arguments"="", "Response"="", "error"={"status"=FALSE, "code"=0, "source"=""}}, "Arguments"=w285, "Response"=w288, "error"=w279) -> (w284:T1)
        n123 = call "Strip CSM name.vi"("CSM name"=w282) -> ("error out"=w280:errorcluster, "CSM name core"=w281:string)  [unwired: 7 in, 2 out]
        n124 = Concatenate Strings(w277, ":" ("string"), w289) -> (w287:string)
        n125 = Merge Errors(w280, w275) -> (w276:errorcluster)
        n126 = disable-structure shown="Enabled" {
          disable-tunnel: w284 -> [w299 _]
          frame Enabled {
            n127 = global write "Global-TestcaseCSM.vi" "response"(w299) -> ()
          }
          frame Disabled {
          }
        }
        n128 = call "CSM - Set Module Attribute.vi"("CSM Name"=w281, "Attribute"=w287, "Value"=w284, "Error In"=w276) -> ("error out"=w286:errorcluster)  [unwired: 8 in, 3 out]
        n129 = call <vilib>:"Add State(s) to Queue__JKI_lib_State_Machine.vi"("State(s) in (\"\")"=w294) -> ("States Out"=w295:string)  [unwired: 14 in]
        n130 = Merge Errors(w286, w279, w292) -> (w291:errorcluster)
      }
      frame "API: Test AsyncMessageWithReply" {
        n131 = call "CSM - Check If Module Exists.vi"("CSM Name"=w313) -> ("error out"=w307:errorcluster, "Exist?"=w308:bool, "CSM Name (Dup)"=w312:string)  [unwired: 8 in]
        n132 = case shown="True" w308 {
          tunnel: w312 -> [_ w316]
          tunnel: [_ w315] -> w309
          frame False {
          }
          frame True {
            n133 = call "uuid.vi"() -> ("UUID"=w317:string)  [unwired: 11 in]
            n134 = call-poly "Build Message with Arguments++.vi"("State With Arguments"="Message", "Arguments (\"\")"=w317, "Target Module (\"\")"=w316) -> ("CSM Message String"=w315:string)  [unwired: 12 in]
          }
        }
        n135 = call <vilib>:"Add State(s) to Queue__JKI_lib_State_Machine.vi"("State(s) in Front (\"\")"=w309, "State(s) in (\"\")"=w310) -> ("States Out"=w311:string)  [unwired: 13 in]
      }
      frame "API: Test AsyncMessageWithReply With Error" {
        n136 = call "CSM - Check If Module Exists.vi"("CSM Name"=w325) -> ("error out"=w319:errorcluster, "Exist?"=w320:bool, "CSM Name (Dup)"=w324:string)  [unwired: 8 in]
        n137 = case shown="True" w320 {
          tunnel: w324 -> [_ w329]
          tunnel: [_ w327] -> w321
          frame False {
          }
          frame True {
            n138 = call "uuid.vi"() -> ("UUID"=w328:string)  [unwired: 11 in]
            n139 = call-poly "Build Message with Arguments++.vi"("State With Arguments"="Message With Error", "Arguments (\"\")"=w328, "Target Module (\"\")"=w329) -> ("CSM Message String"=w327:string)  [unwired: 12 in]
          }
        }
        n140 = call <vilib>:"Add State(s) to Queue__JKI_lib_State_Machine.vi"("State(s) in Front (\"\")"=w321, "State(s) in (\"\")"=w322) -> ("States Out"=w323:string)  [unwired: 13 in]
      }
      frame "API: Test AsyncMessageWithoutReply" {
        n141 = call "CSM - Check If Module Exists.vi"("CSM Name"=w337) -> ("error out"=w331:errorcluster, "Exist?"=w332:bool, "CSM Name (Dup)"=w336:string)  [unwired: 8 in]
        n142 = case shown="True" w332 {
          tunnel: w336 -> [_ w342]
          tunnel: [_ w340] -> w333
          frame False {
          }
          frame True {
            n143 = call-poly "Build Message with Arguments++.vi"("State With Arguments"="AsyncMessageWithoutReply", "Arguments (\"\")"="123456789" ("Arguments (\"\")"), "Target Module (\"\")"=w342) -> ("CSM Message String"=w340:string)  [unwired: 12 in]
          }
        }
        n144 = call <vilib>:"Add State(s) to Queue__JKI_lib_State_Machine.vi"("State(s) in Front (\"\")"=w333, "State(s) in (\"\")"=w334) -> ("States Out"=w335:string)  [unwired: 13 in]
      }
      frame "API: Test AsyncMessageWithoutReply via API" {
        n145 = call "CSM - Check If Module Exists.vi"("CSM Name"=w351) -> ("error out"=w346:errorcluster, "Exist?"=w347:bool, "CSM Name (Dup)"=w350:string)  [unwired: 8 in]
        n146 = case shown="True" w347 {
          tunnel: w350 -> [_ w354]
          tunnel: w345 -> [_ w357]
          tunnel: [_ w353] -> w343
          frame False {
          }
          frame True {
            n147 = call "CSM - Wait and Post Message.vi"("State"="AsyncMessageWithoutReply" ("State With Arguments"), "Current Module (\"\" to Generate an ID)"=w357, "Arguments (\"\")"="123456789" ("Arguments (\"\")"), "Target Module"=w354) -> ("error out"=w353:errorcluster)  [unwired: 11 in]
          }
        }
        n148 = call <vilib>:"Add State(s) to Queue__JKI_lib_State_Machine.vi"("State(s) in (\"\")"=w348) -> ("States Out"=w349:string)  [unwired: 14 in]
        n149 = Merge Errors(w343, w346) -> (w344:errorcluster)
      }
      frame "API: Test Argument" {
        n150 = call "uuid.vi"() -> ("UUID"=w363:string)  [unwired: 11 in]
        n151 = call "CSM - Convert HexStr to Data.vi"("HEX String"=w367) -> ("Variant"=w365:variant, "error out"=w366:errorcluster)  [unwired: 7 in]
        n152 = Bundle("", "UUID"=w363) -> (w361:cluster{string, "UUID":string})  [unwired: 1 in]
        n153 = Variant To Data(error in=w366, type=w361, Variant=w365) -> (data=w360:cluster{string, "UUID":string}, error out=w364:errorcluster)
        n154 = Unbundle(w360) -> (w359:string, "UUID"=w358:string)
        n155 = call "CSM - Check If Module Exists.vi"("Error In"=w364, "CSM Name"=w359) -> ("error out"=w368:errorcluster, "Exist?"=w369:bool, "CSM Name (Dup)"=w373:string)  [unwired: 7 in]
        n156 = case shown="True" w369 {
          tunnel: w373 -> [_ w377]
          tunnel: [_ w376] -> w370
          tunnel: w358 -> [_ w375]
          frame False {
          }
          frame True {
            n157 = call "Build Synchronous Message with Arguments.vi"("State With Arguments"="ArgumentTest", "Arguments (\"\")"=w375, "Target Module (\"\")"=w377) -> ("CSM Message String"=w376:string)  [unwired: 12 in]
          }
        }
        n158 = call <vilib>:"Add State(s) to Queue__JKI_lib_State_Machine.vi"("State(s) in Front (\"\")"=w370, "State(s) in (\"\")"=w371) -> ("States Out"=w372:string)  [unwired: 13 in]
      }
      frame "API: Test Response With Error" {
        n159 = call "CSM - Check If Module Exists.vi"("CSM Name"=w385) -> ("error out"=w379:errorcluster, "Exist?"=w380:bool, "CSM Name (Dup)"=w384:string)  [unwired: 8 in]
        n160 = case shown="True" w380 {
          tunnel: w384 -> [_ w388]
          tunnel: [_ w387] -> w381
          frame False {
          }
          frame True {
            n161 = call "uuid.vi"() -> ("UUID"=w389:string)  [unwired: 11 in]
            n162 = call "Build Synchronous Message with Arguments.vi"("State With Arguments"="Response With Error", "Arguments (\"\")"=w389, "Target Module (\"\")"=w388) -> ("CSM Message String"=w387:string)  [unwired: 12 in]
          }
        }
        n163 = call <vilib>:"Add State(s) to Queue__JKI_lib_State_Machine.vi"("State(s) in Front (\"\")"=w381, "State(s) in (\"\")"=w382) -> ("States Out"=w383:string)  [unwired: 13 in]
      }
      frame "API: Test MacroWithSubMessages" {
        n164 = call <vilib>:"Build State String with Arguments__JKI_lib_State_Machine.vi"("Arguments (\"\")"=w392, "State"="Macro: Test MacroWithSubMessages") -> ("State with Arguments"=w391:string)  [unwired: 4 in]
        n165 = call <vilib>:"Add State(s) to Queue__JKI_lib_State_Machine.vi"("State(s) in Front (\"\")"=w391, "State(s) in (\"\")"=w395) -> ("States Out"=w394:string)  [unwired: 13 in]
      }
      frame "API: Test MacroWithSubAndPostMessages" {
        n166 = call <vilib>:"Build State String with Arguments__JKI_lib_State_Machine.vi"("Arguments (\"\")"=w399, "State"="Macro: Test MacroWithSubAndPostMessages") -> ("State with Arguments"=w398:string)  [unwired: 4 in]
        n167 = call <vilib>:"Add State(s) to Queue__JKI_lib_State_Machine.vi"("State(s) in Front (\"\")"=w398, "State(s) in (\"\")"=w402) -> ("States Out"=w401:string)  [unwired: 13 in]
      }
      frame "API: Test MacroWithNonLocalSubMessages" {
        n168 = call <vilib>:"Build State String with Arguments__JKI_lib_State_Machine.vi"("Arguments (\"\")"=w406, "State"="Macro: TestMacroWithNonLocalSubMessages") -> ("State with Arguments"=w405:string)  [unwired: 4 in]
        n169 = call <vilib>:"Add State(s) to Queue__JKI_lib_State_Machine.vi"("State(s) in Front (\"\")"=w405, "State(s) in (\"\")"=w409) -> ("States Out"=w408:string)  [unwired: 13 in]
      }
      frame "API: Test Register State" {
        n170 = call <vilib>:"Build State String with Arguments__JKI_lib_State_Machine.vi"("Arguments (\"\")"=w413, "State"="Register State") -> ("State with Arguments"=w412:string)  [unwired: 4 in]
        n171 = call <vilib>:"Add State(s) to Queue__JKI_lib_State_Machine.vi"("State(s) in Front (\"\")"=w412, "State(s) in (\"\")"=w416) -> ("States Out"=w415:string)  [unwired: 13 in]
      }
      frame "API: Test Register Status" {
        n172 = call <vilib>:"Build State String with Arguments__JKI_lib_State_Machine.vi"("Arguments (\"\")"=w420, "State"="Register Status") -> ("State with Arguments"=w419:string)  [unwired: 4 in]
        n173 = call <vilib>:"Add State(s) to Queue__JKI_lib_State_Machine.vi"("State(s) in Front (\"\")"=w419, "State(s) in (\"\")"=w423) -> ("States Out"=w422:string)  [unwired: 13 in]
      }
      frame "API: Local Registration" {
        # "Test Status @ From >> Handler Message @ To -><register>"
        n174 = call "Strip CSM name.vi"("CSM name"=w431) -> ("error out"=w429:errorcluster, "CSM name core"=w426:string)  [unwired: 7 in, 2 out]
        n175 = call-poly "Build Message with Arguments++.vi"("Target CSM"=w427, "Source CSM (* as Default)"=w426, "Status"="Test Status", "API (If \"\", Same As \"Status\")"="Handler Message") -> ("CSM Message String"=w428:string)  [unwired: 11 in]
        n176 = call <vilib>:"Add State(s) to Queue__JKI_lib_State_Machine.vi"("State(s) in Front (\"\")"=w428, "State(s) in (\"\")"=w435) -> ("States Out"=w434:string)  [unwired: 13 in]
      }
      frame "API: Local Unregistration" {
        # "Test Status @ From >> Handler Message @ To -><unregister>"
        n177 = call "Strip CSM name.vi"("CSM name"=w441) -> ("error out"=w439:errorcluster, "CSM name core"=w436:string)  [unwired: 7 in, 2 out]
        n178 = call-poly "Build Message with Arguments++.vi"("Target CSM"=w437, "Source CSM (* as Default)"=w436, "Status"="Test Status", "API (* as Default)"="Handler Message") -> ("CSM Message String"=w438:string)  [unwired: 11 in]
        n179 = call <vilib>:"Add State(s) to Queue__JKI_lib_State_Machine.vi"("State(s) in Front (\"\")"=w438, "State(s) in (\"\")"=w445) -> ("States Out"=w444:string)  [unwired: 13 in]
      }
      frame "API: Local Registration via API" {
        # "Test Status @ From >> Handler Message @ To -><register>"
        n180 = call "Strip CSM name.vi"("CSM name"=w452) -> ("error out"=w451:errorcluster, "CSM name core"=w447:string)  [unwired: 7 in, 2 out]
        n181 = call "CSM - Register Status Change.vi"("CSM Name"=w446, "Source CSM Name (* as Default)"=w447, "Status"="Test Status", "Response Message (If \"\", Same as Source Message)"="Handler Message", "Error In"=w451) -> ("error out"=w450:errorcluster)  [unwired: 9 in, 1 out]
        n182 = call <vilib>:"Add State(s) to Queue__JKI_lib_State_Machine.vi"("State(s) in (\"\")"=w455) -> ("States Out"=w454:string)  [unwired: 14 in]
      }
      frame "API: Local Unregistration via API" {
        # "Test Status @ From >> Handler Message @ To -><unregister>"
        n183 = call "Strip CSM name.vi"("CSM name"=w462) -> ("error out"=w461:errorcluster, "CSM name core"=w457:string)  [unwired: 7 in, 2 out]
        n184 = call "CSM - Unregister Status Change.vi"("CSM Name"=w456, "Source CSM Name (* as Default)"=w457, "Status"="Test Status", "Response Message (\"*\" as Default)"="Handler Message", "Error In"=w461) -> ("error out"=w460:errorcluster)  [unwired: 9 in, 1 out]
        n185 = call <vilib>:"Add State(s) to Queue__JKI_lib_State_Machine.vi"("State(s) in (\"\")"=w465) -> ("States Out"=w464:string)  [unwired: 14 in]
      }
      frame "API: API2" {
        # "#CSM API Example\nCopy/Rename this case for your own API"
        # "unpack Hex String  to Variant\nif complex parameter is needed."
        n186 = call "CSM - Convert HexStr to Data.vi"("HEX String"=w467) -> ()  [unwired: 7 in, 2 out]
        n187 = disable-structure shown="Disabled" {
          disable-tunnel: [w470 "API2 Response"] -> w466
          frame Disabled {
            # "pack variant to hexstr \nif complex response is needed."
            # "complex Response"
            n188 = call "CSM - Convert Data to HexStr.vi"() -> ("HEX String (0-9,A-F)"=w470:string)  [unwired: 9 in]
          }
          frame Enabled {
          }
        }
      }
      frame "---------- Action ----------" {
        # "#CSM \"Category Seperator\"\nDo not put any code in this frame."
        n189 = call <vilib>:"Add State(s) to Queue__JKI_lib_State_Machine.vi"("State(s) in (\"\")"=w474) -> ("States Out"=w473:string)  [unwired: 14 in]
      }
      frame "Action: action1" {
        # "#CSM \"Internal State\"\nThis category is used for holding internal states"
        n190 = call <vilib>:"Add State(s) to Queue__JKI_lib_State_Machine.vi"("State(s) in (\"\")"=w477) -> ("States Out"=w476:string)  [unwired: 14 in]
      }
      frame "Register State" {
        n191 = call <vilib>:"Build State String with Arguments__JKI_lib_State_Machine.vi"("Arguments (\"\")"=w479, "State"="Register Status" ("State(s) in Front (\"\")")) -> ("State with Arguments"=w478:string)  [unwired: 4 in]
        n192 = call <vilib>:"Add State(s) to Queue__JKI_lib_State_Machine.vi"("State(s) in Front (\"\")"=w478, "State(s) in (\"\")"=w483) -> ("States Out"=w482:string)  [unwired: 13 in]
      }
      frame "Register Status" {
        n193 = call <vilib>:"Build State String with Arguments__JKI_lib_State_Machine.vi"("Arguments (\"\")"=w484, "State"="Test Status") -> ("State with Arguments"=w486:string)  [unwired: 4 in]
        n194 = call "CSM - Broadcast Status Change.vi"("Status With Arguments"=w486, "State Queue"=w488) -> ("Remaining States"=w485:string)  [unwired: 13 in]
      }
      frame "Message" {
      }
      frame "SubMessage1" {
      }
      frame "SubMessage2" {
      }
      frame "SubMessage3" {
        n195 = call "Strip CSM name.vi"("CSM name"=w508) -> ("error out"=w506:errorcluster, "CSM name core"=w507:string)  [unwired: 7 in, 2 out]
        n196 = call "CSM - Set Module Attribute.vi"("CSM Name"=w507, "Attribute"=w505, "Value"=w504, "Error In"=w506) -> ("error out"=w502:errorcluster)  [unwired: 8 in, 3 out]
        n197 = Merge Errors(w502, w511) -> (w503:errorcluster)
      }
      frame "PostMessage1" {
      }
      frame "Message With Error" {
        n198 = Merge Errors(errorcluster {"status"=TRUE, "code"=1234567898, "source"="Simulated Error\nwill be sent to Response case"} ("error out"), w517) -> (w516:errorcluster)
      }
      frame "Response With Error" {
        n199 = Merge Errors(errorcluster {"status"=TRUE, "code"=1234567898, "source"="Simulated Error"} ("error out"), w523) -> (w522:errorcluster)
      }
      frame "ArgumentTest" {
        n200 = call "Strip CSM name.vi"("CSM name"=w534) -> ("error out"=w531:errorcluster, "CSM name core"=w533:string)  [unwired: 7 in, 2 out]
        n201 = call "CSM Set Module Attribute.vim"("CSM Name"=w533, "Attribute"=w530, "Value"=w532, "Error In"=w531) -> ("error out"=w528:errorcluster)  [unwired: 8 in, 3 out]
        n202 = Merge Errors(w528, w537) -> (w529:errorcluster)
      }
      frame "AsyncMessageWithoutReply" {
        # "123456789 string constant"
        n203 = call "Strip CSM name.vi"("CSM name"=w542) -> ("error out"=w540:errorcluster, "CSM name core"=w541:string)  [unwired: 7 in, 2 out]
        n204 = call "CSM - Set Module Attribute.vi"("CSM Name"=w541, "Attribute"=w543, "Value"=w544, "Error In"=w540) -> ("error out"=w538:errorcluster)  [unwired: 8 in, 3 out]
        n205 = Merge Errors(w538, w547) -> (w539:errorcluster)
      }
      frame "Handler Message" {
        n206 = call "Strip CSM name.vi"("CSM name"=w554) -> ("error out"=w552:errorcluster, "CSM name core"=w553:string)  [unwired: 7 in, 2 out]
        n207 = call "CSM Set Module Attribute.vim"("CSM Name"=w553, "Attribute"=w549, "Value"=w548, "Error In"=w552) -> ("error out"=w550:errorcluster)  [unwired: 8 in, 3 out]
        n208 = Merge Errors(w550, w557) -> (w551:errorcluster)
      }
    }
  }
